vi "Add Measurement.vi"(7 "overwrite?":bool=TRUE, 9 "error in (no error)":errorcluster, 10 "entry":cluster{"key":string, "value":variant}, 11 "Properties":refnum<class "Properties.lvclass">) -> (1 "error out":errorcluster, 3 "Properties":refnum<class "Properties.lvclass">)   [LabVIEW 2013, in "Caraya.lvlib" / "Properties.lvclass"]
uses:
  Properties.lvclass
  Properties.lvclass/Properties.ctl
  Test Manager Message Measurement/TestManagerMsg.Measurement.lvclass
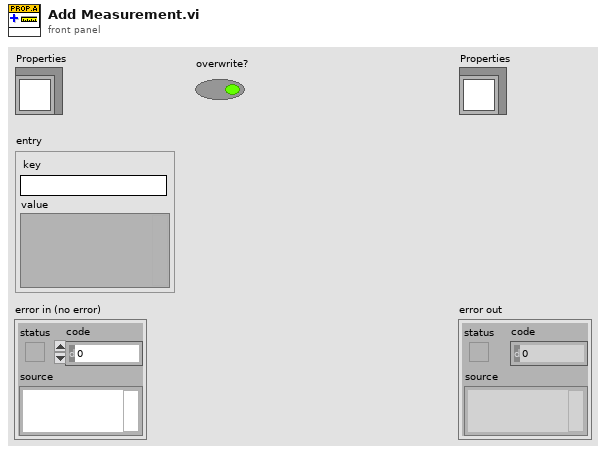
[diagram p1: front panel]
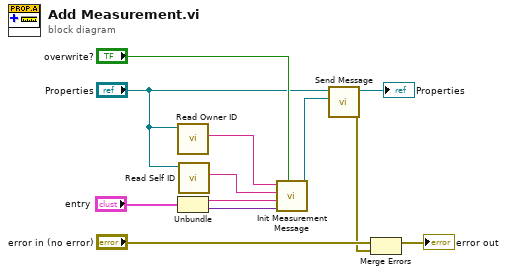
[diagram p0: block diagram]
diagram:
  n1 = call "Read Owner ID.vi"("Properties in"="Properties") -> ("owner-id"=w5:string)  [unwired: 9 in, 1 out]
  n2 = Unbundle("entry") -> ("key"=w8:string, "value"=w7:variant)
  n3 = call "Read Self ID.vi"("Properties in"="Properties") -> ("self-id"=w6:string)  [unwired: 9 in, 1 out]
  n4 = call "Init Measurement Message.vi"("overwrite?"="overwrite?", "Value"=w7, "name"=w8, "self-id"=w6, "owner-id"=w5) -> ("Message"=w1:refnum<class "TestManagerMsg.lvclass">)  [unwired: 6 in]
  n5 = call "Send Message.vi"("TestManagerMsg"=w1, "Properties in"="Properties") -> ("error out"=w3:errorcluster, "Properties out"=→"Properties":refnum<class "Properties.lvclass">)  [unwired: 8 in]
  n6 = Merge Errors("error in (no error)", w3) -> (→"error out":errorcluster)
